vi "SendOneFrame.vi"(0 "类型":u32(ring)=4 items=["PCI5121"=1, "PCI9810"=2, "USBCAN1"=3, "USBCAN2"=4, "PCI9820"=5, "CAN232"=6, "PCI5110"=7, "CANLite(mini)"=8, "ISA9620"=9, "ISA5420"=10, "PC104CAN"=11, "CANET"=17, "DNP9810"=13, "USBCAN-E-U"=20, "USBCAN-2E-U"=21], 1 "设备索引":u32(ring) items=["0", "1", "2", "3", "4", "5", "6", "7", "8", "9", "10", "11", "12", "13", "14", "15", ""], 4 "CAN路数":u32(ring) items=["0", "1"], 7 "ID":u32 format="%x", 9 "DataLen":u8, 11 "ExternFlag":u8, 13 "数组":u8[](array[numeric])) -> (14 "发送状态":bool)   [LabVIEW 2018]
uses:
  ControlCAN/64/ControlCAN.dll
panel:
  out "VCI_CAN_OBJ_T":T1 {"ID" format="%x"}
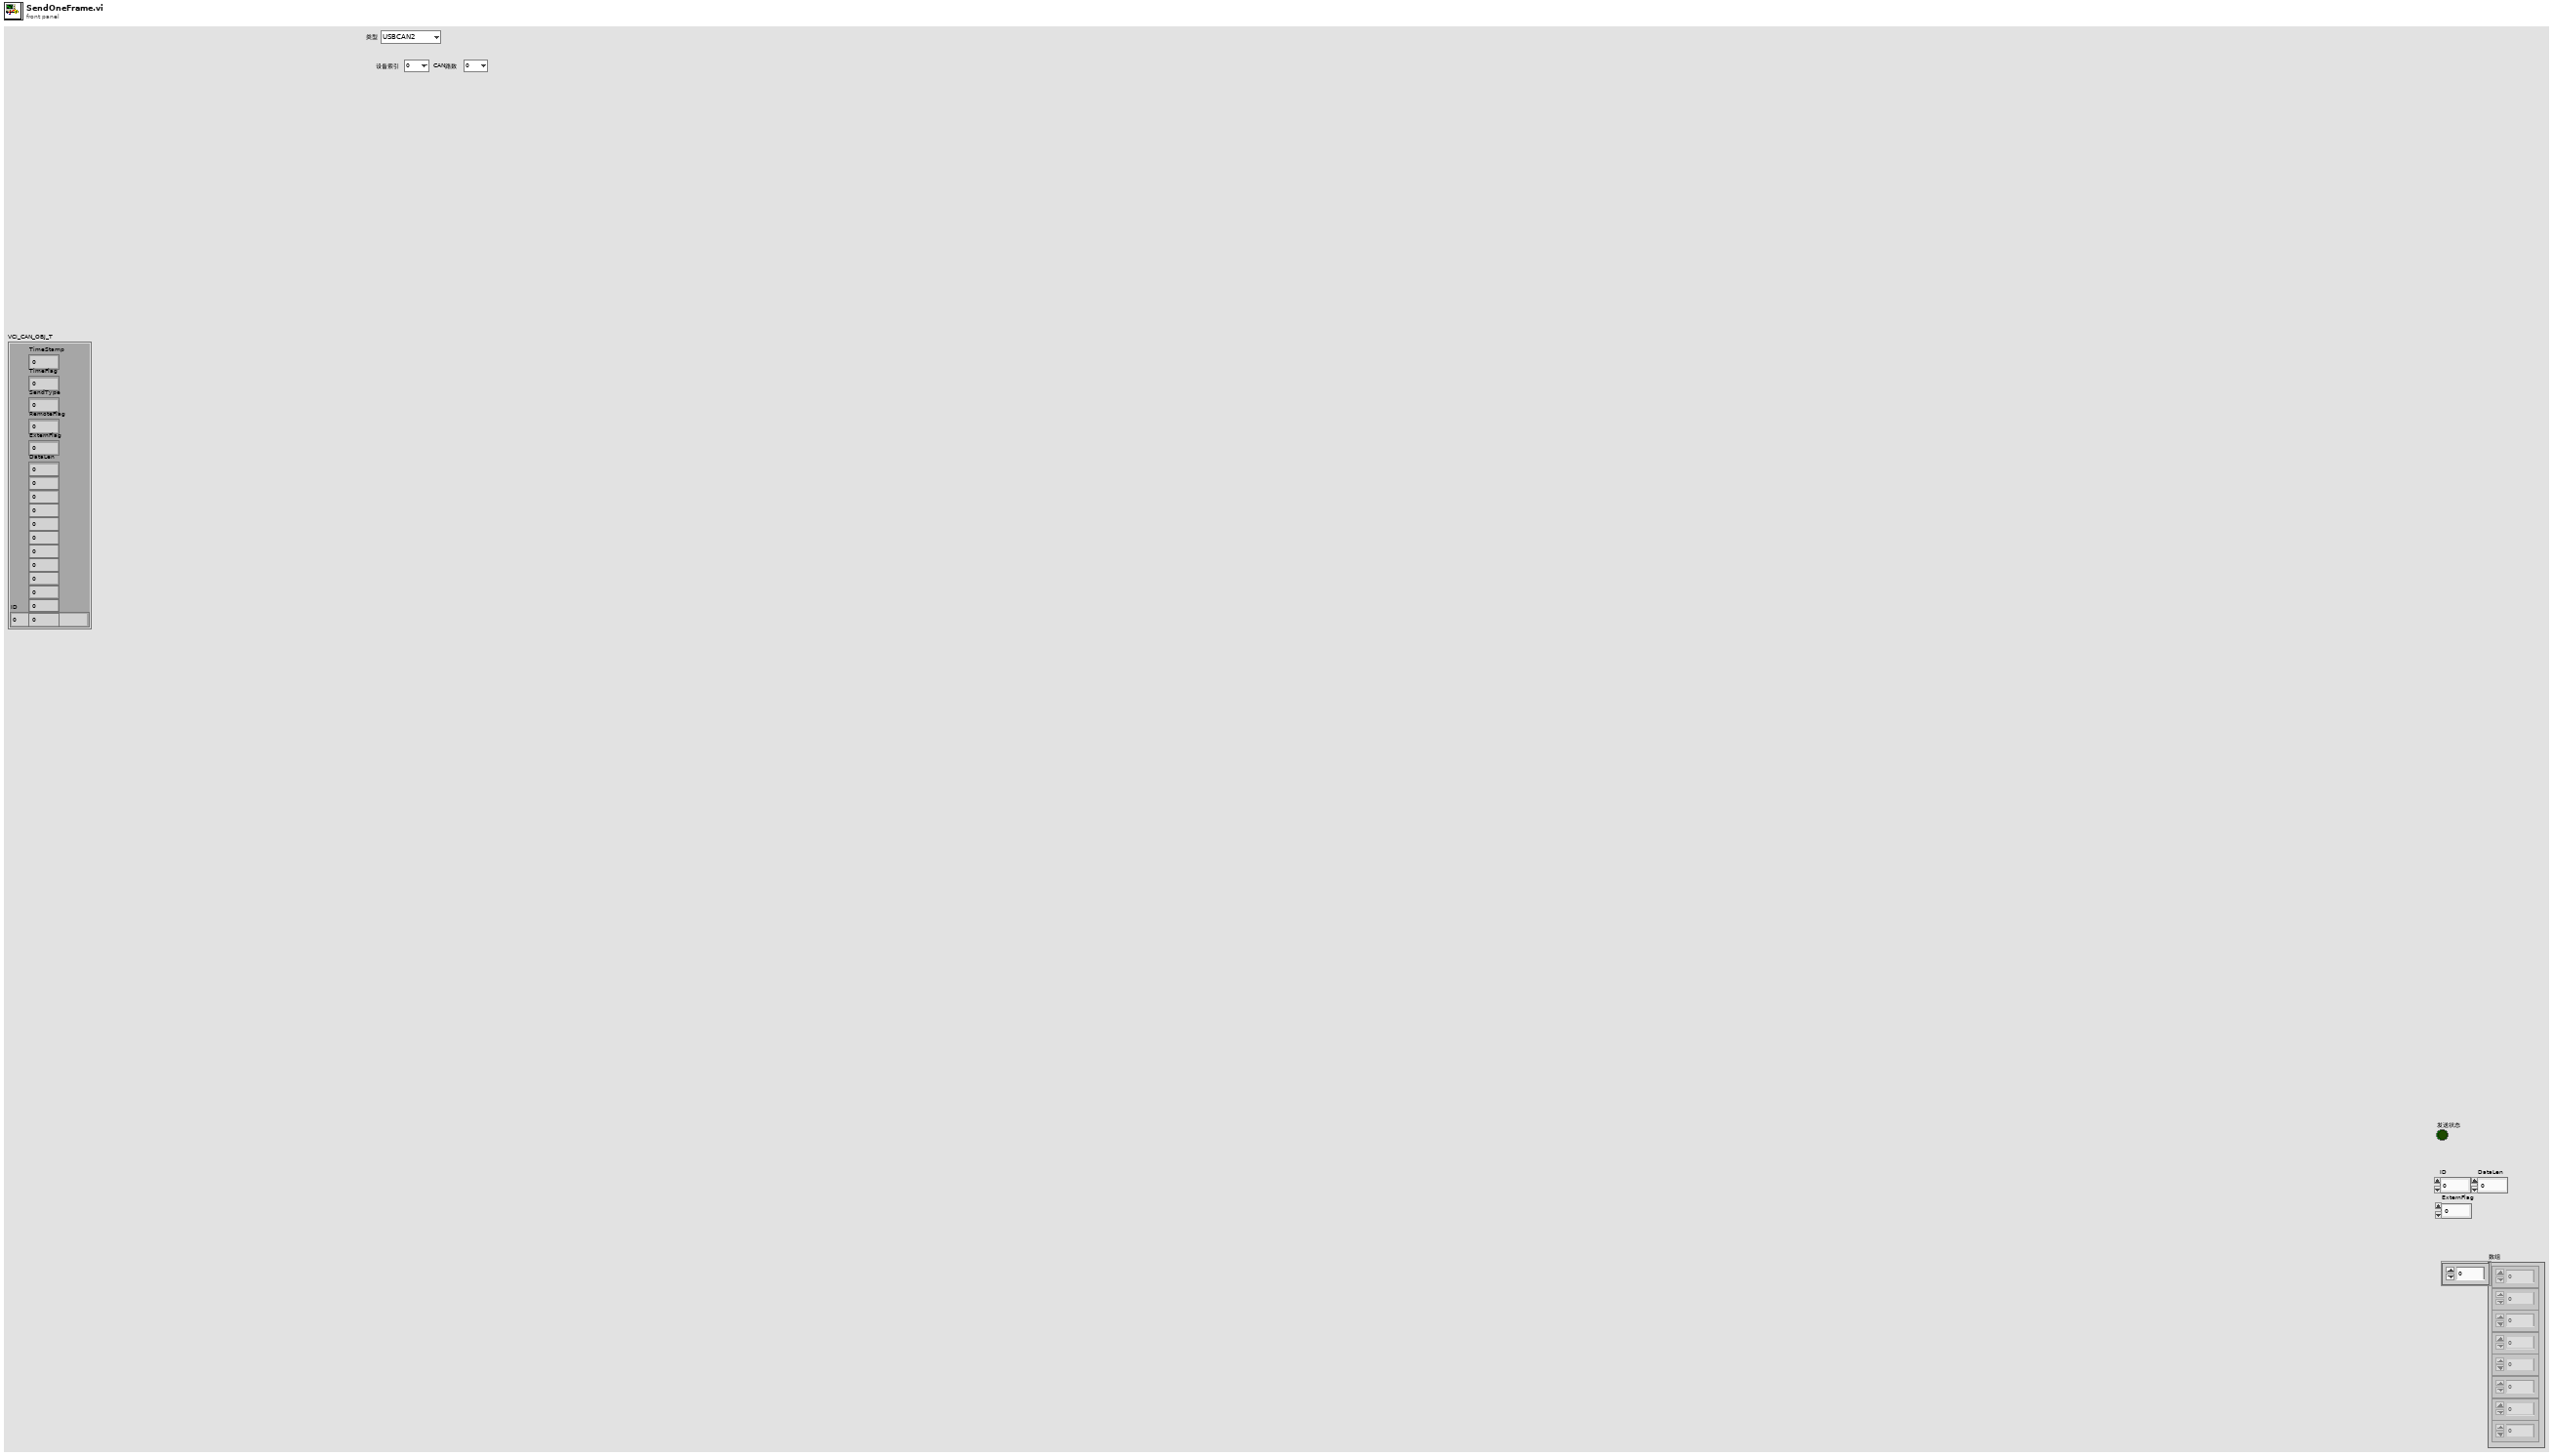
[diagram p1: front panel]
types:
  T1 = cluster{"ID":u32, "TimeStamp":u32, "TimeFlag":u8, "SendType":u8, "RemoteFlag":u8, "ExternFlag":u8, "DataLen":u8, u8, u8, u8, u8, u8, u8, u8, u8, u8, u8, u8}
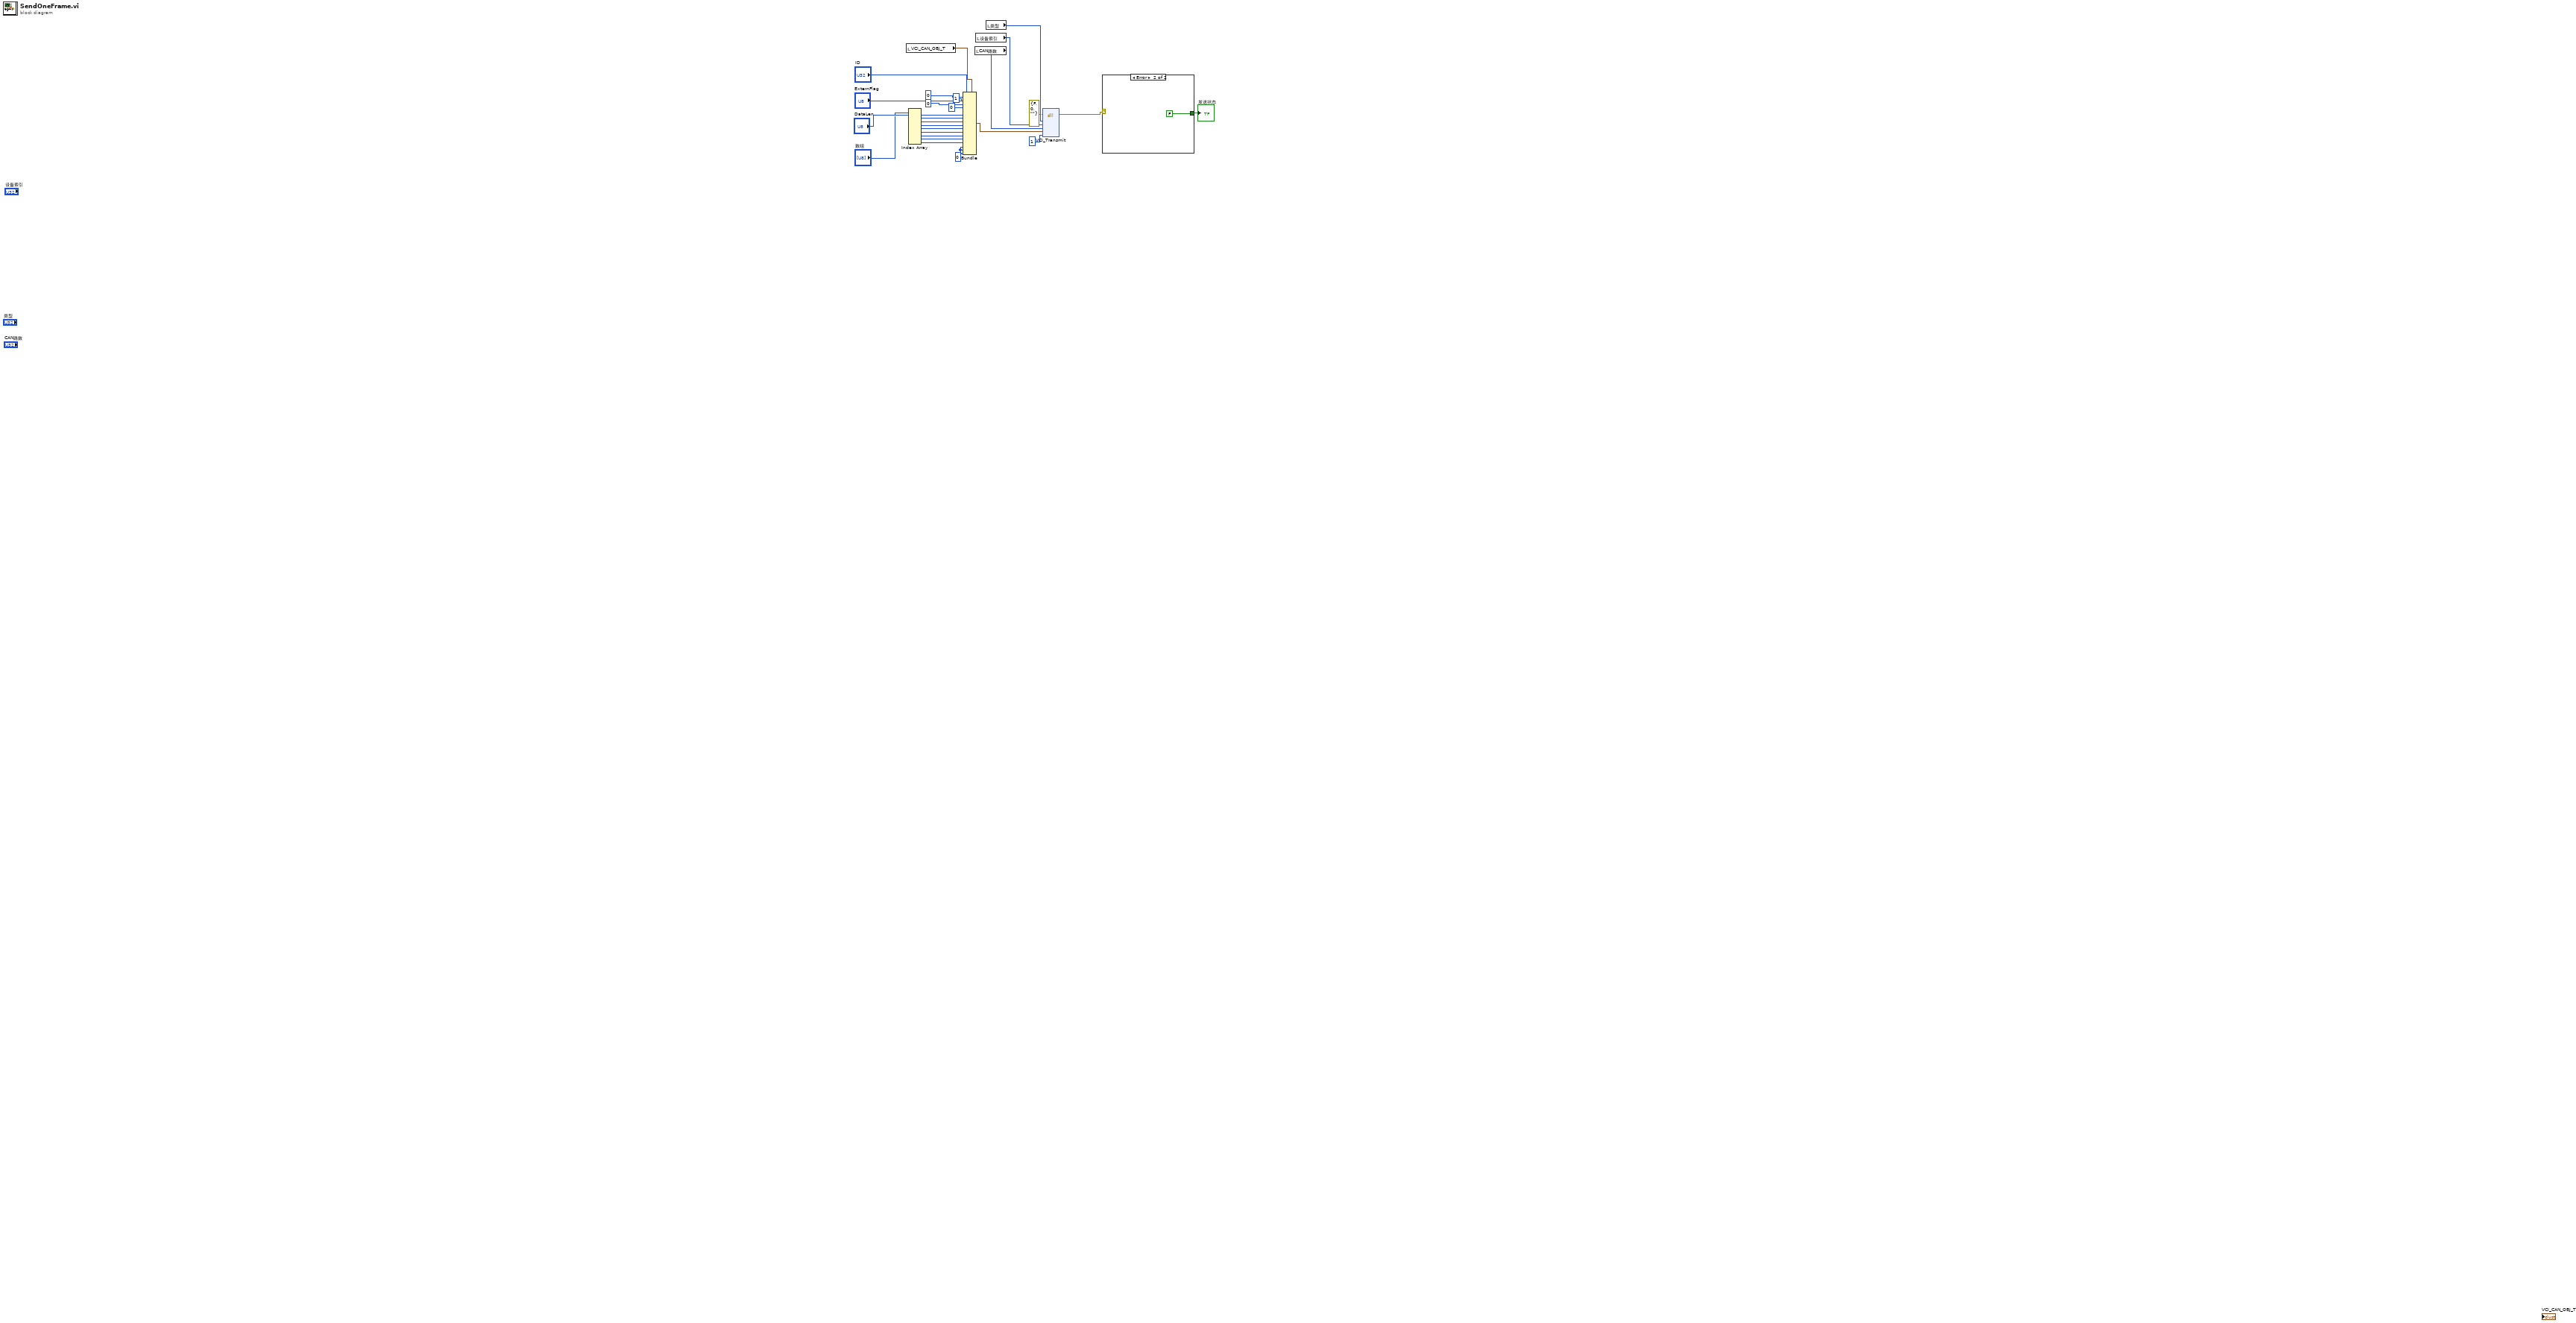
[diagram p0: block diagram]
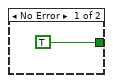
[diagram p2: hidden frame]
diagram:
  w17 = u8 0 ("元素")
  n1 = local read "VCI_CAN_OBJ_T"() -> (w21:T1)
  n2 = Index Array(array="数组") -> (element #1=w11:u8, element #2=w10:u8, element #3=w9:u8, element #4=w8:u8, element #5=w7:u8, element #6=w6:u8, element #7=w5:u8, element #8=w4:u8)  [unwired: 8 in]
  n3 = Bundle(cluster=w21, "ID"="ID", "TimeStamp"=u8 0 ("RemoteFlag"), "TimeFlag"=u8 1, "SendType"=u8 0 ("DataLen"), "RemoteFlag"=u8 0, "ExternFlag"="ExternFlag", "DataLen"="DataLen", w11, w10, w9, w8, w7, w6, w5, w4, w17, w17, w17) -> (w25:T1)
  n4 = local read "CAN路数"() -> (w22:u32)
  n5 = local read "设备索引"() -> (w23:u32)
  n6 = local read "类型"() -> (w24:u32)
  n7 = dll-call lib="C:/Users/Administrator/Desktop/AutoTest_TestStand/trunk/AutoTest_TestStand/Driver/ZlgCan/ControlCAN/64/ControlCAN.dll" fn="VCI_Transmit"(error in=errorcluster {"status"=FALSE, "code"=0, "source"=""} ("错误输入（无错误）"), "DeviceType"=w24, "DeviceInd"=w23, "CANInd"=w22, "pSend"=w25, "Len"=u32 1) -> (error out=w2:errorcluster)  [unwired: 4 in, 5 out]
  n8 = case shown="Error" w2 {
    tunnel: [TRUE FALSE] -> w1
    frame No Error {
    }
    frame Error {
    }
  }
  "发送状态" <- w1
